vi "SubcribeStripHeader.vi"(10 "New Data":string, 11 "Data Input":string) -> (1 "Headers":string, 3 "Data Output":string)   [LabVIEW 2015]
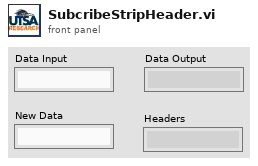
[diagram p1: front panel]
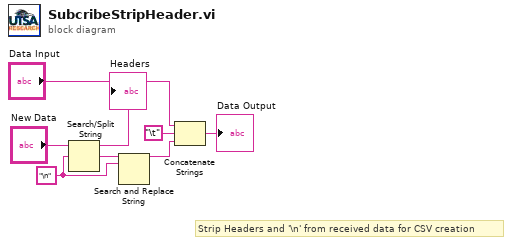
[diagram p0: block diagram]
diagram:
  w7 = "\n" ("search string/char (-)")
  # "Strip Headers and '\\n' from received data for CSV creation"
  n1 = Search/Split String(string="New Data", search string/char (-)=w7) -> (substring before match=→"Headers":string, match + rest of string=w6:string)  [unwired: 1 in, 1 out]
  n2 = Search and Replace String(input string=w6, search string=w7) -> (result string=w8:string)  [unwired: 6 in, 3 out]
  n3 = Concatenate Strings("Data Input", "\t", w8) -> (→"Data Output":string)
